vi "add_InertiaStamped.vi"(5 "Inertia":T1, 6 "Cluster":cluster{"frame_id":string, "reset seq?":bool}, 7 "msg in":string) -> (3 "msg out":string)   [LabVIEW 2012]
doc: "Flattens an inertia stamped into a message"
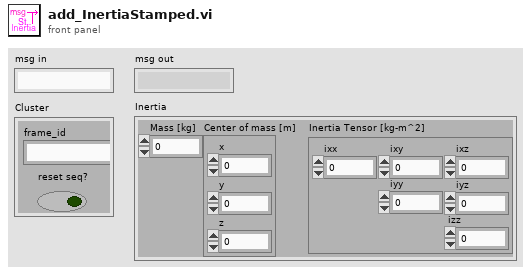
[diagram p1: front panel]
types:
  T1 = cluster{"Mass [kg]":dbl, "Center of mass [m]":cluster{"x":dbl, "y":dbl, "z":dbl}, "Inertia Tensor [kg-m^2]":cluster{"ixx":dbl, "ixy":dbl, "ixz":dbl, "iyy":dbl, "iyz":dbl, "izz":dbl}}
  T2 = cluster{"ixx":dbl, "ixy":dbl, "ixz":dbl, "iyy":dbl, "iyz":dbl, "izz":dbl}
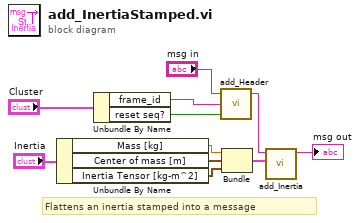
[diagram p0: block diagram]
diagram:
  # "Flattens an inertia stamped into a message"
  n1 = Unbundle By Name("Inertia") -> ("Mass [kg]"=w7:dbl, "Center of mass [m]"=w6:cluster{"x":dbl, "y":dbl, "z":dbl}, "Inertia Tensor [kg-m^2]"=w5:T2)
  n2 = Unbundle By Name("Cluster") -> ("frame_id"=w2:string, "reset seq?"=w1:bool)
  n3 = call <userlib>:"add_Header.vi"("reset seq?"=w1, "frame_id"=w2, "msg in"="msg in") -> ("msg out"=w10:string)  [unwired: 2 in]
  n4 = Bundle("Mass [kg]"=w7, "Center of mass [m]"=w6, "Inertia Tensor [kg-m^2]"=w5) -> (w4:T1)  [unwired: 1 in]
  n5 = call <userlib>:"add_Inertia.vi"("Inertia"=w4, "msg in"=w10) -> ("msg out"=→"msg out":string)  [unwired: 5 in]
